vi "C37 Get PMU Real Data.vi"(7 "Array Lengths":T1, 10 "pseudoPdcId":i32, 11 "pmuIndex":i32) -> (1 "Digital Values":bool[](array[boolean]), 2 "Analog Values":sgl[](array[numeric]), 3 "Phasor Values":csg[](array[numeric]), 4 "Frequency":sgl, 5 "function return":i32, 6 "Delta Frequency":sgl)   [LabVIEW 2012]
doc: "STRONGRIDIEEEC37118DLL_API int __cdecl getPmuRealDataLabview(noArraysPmuDataFrame* rd, PmuStatus* status,\n uint16_t PhasorArrayLength, float* phasorValueReal, float* phasorValueImaginary,\n uint16_t AnalogArrayLength, float* analogValueArr,\n uint16_t DigitalArrayLength, uint8_t* digitalValueArr,\n int32_t pseudoPdcId, int32_t pmuIndex);\n\nSTRONGRIDIEEEC37118DLL_API int __cdecl getPmuRealDataLabview(noArraysPmuDataFrame* rd, PmuStatus* status,\n uint16_t PhasorArrayLength, float* phasorValueReal, float* phasorValueImaginary,\n uint16_t AnalogArrayLength, float* analogValueArr,\n uint16_t DigitalArrayLength, uint8_t* digitalValueArr,\n int32_t pseudoPdcId, int32_t pmuIndex);"
uses:
  Auto Generated/StrongridDLL.dll
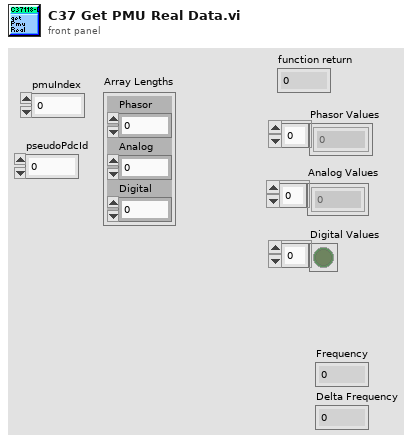
[diagram p1: front panel]
types:
  T1 = cluster{"Phasor":i32, "Analog":i32, "Digital":i32}
  T2 = cluster{"dataErrorCode":u8, "pmuSyncFlag":u8, "pmuDataSortingFlag":u8, "pmuTriggerFlag":u8, "configChangeFlag":u8, "dataModifiedFlag":u8, "timeQualityCode":u8, "unlockTimeCode":u8, "triggerReasonCode":u8}
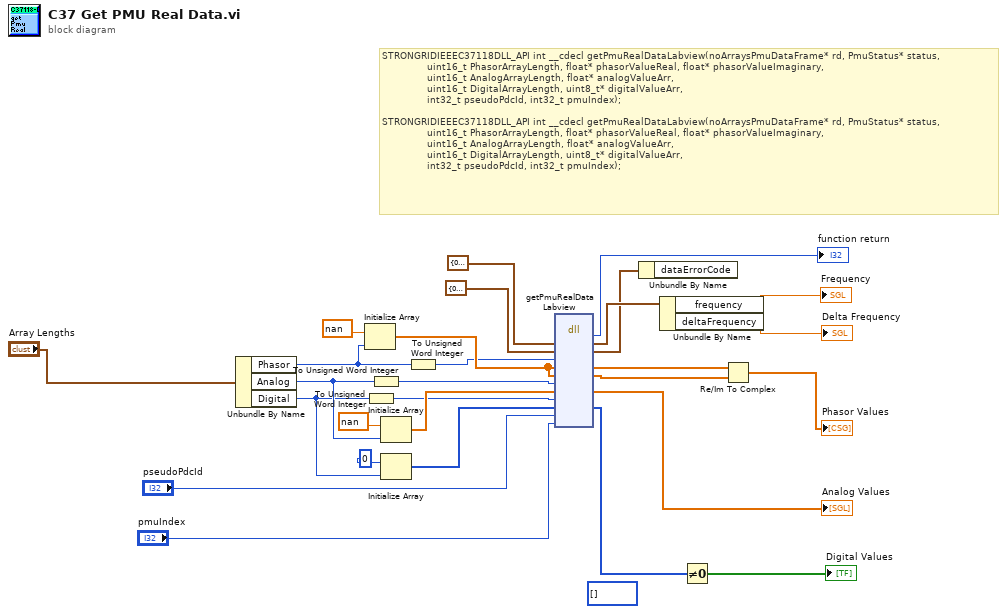
[diagram p0: block diagram]
diagram:
  (unwired) i8[] [] ("digitalValueArr")
  # "STRONGRIDIEEEC37118DLL_API int __cdecl getPmuRealDataLabview(noArraysPmuDataFrame* rd, PmuStatus* status,\n               uint16_t PhasorArrayLength, float* phasorValueReal, float* phasorValueImaginary,\n               uint16_t AnalogArrayLength, float* analogValueArr,\n               uint16_t DigitalArrayLength, uint8_t* digitalValueArr,\n               int32_t pseudoPdcId, int32_t pmuIndex);\n\nSTRONGRIDIEEEC37118DLL_API int __cdecl getPmuRealDataLabview(noArraysPmuDataFrame* rd, PmuStatus* status,\n\t\t\t\t\t\t\t\t\t\t\t\t\t\t\tuint16_t PhasorArrayLength, float* phasorValueReal, float* phasorValueImaginary,\n\t\t\t\t\t\t\t\t\t\t\t\t\t\t\tuint16_t AnalogArrayLength, float* analogValueArr,\n\t\t\t\t\t\t\t\t\t\t\t\t\t\t\tuint16_t DigitalArrayLength, uint8_t* digitalValueArr,\n\t\t\t\t\t\t\t\t\t\t\t\t\t\t\tint32_t pseudoPdcId, int32_t pmuIndex);"
  n1 = Unbundle By Name("Array Lengths") -> ("Phasor"=w12:i32, "Analog"=w8:i32, "Digital"=w5:i32)
  n2 = Initialize Array(sgl nan ("frequency"), w12) -> (w10:sgl[])
  n3 = To Unsigned Word Integer(number=w5) -> (unsigned 16bit integer=w1:u16)
  n4 = To Unsigned Word Integer(number=w8) -> (unsigned 16bit integer=w2:u16)
  n5 = Initialize Array(sgl nan ("frequency"), w8) -> (w7:sgl[])
  n6 = Initialize Array(i8 0 ("frequency"), w5) -> (w4:i8[])
  n7 = To Unsigned Word Integer(number=w12) -> (unsigned 16bit integer=w3:u16)
  n8 = dll-call lib="C:/dev/c37118-dll/labview/vi/Auto Generated/StrongridDLL.*" fn="getPmuRealDataLabview"("rd"=cluster{"frequency":sgl, "deltaFrequency":sgl} {"frequency"=0.0, "deltaFrequency"=0.0}, "status"=T2 {"dataErrorCode"=0, "pmuSyncFlag"=0, "pmuDataSortingFlag"=0, "pmuTriggerFlag"=0, "configChangeFlag"=0, "dataModifiedFlag"=0, "timeQualityCode"=0, "unlockTimeCode"=0, "triggerReasonCode"=0}, "PhasorArrayLength"=w3, "phasorValueReal"=w10, "phasorValueImaginary"=w10, "AnalogArrayLength"=w2, "analogValueArr"=w7, "DigitalArrayLength"=w1, "digitalValueArr"=w4, "pseudoPdcId"="pseudoPdcId", "pmuIndex"="pmuIndex") -> ("return type"=→"function return":i32, "rd"=w22:cluster{"frequency":sgl, "deltaFrequency":sgl}, "status"=w19:T2, "phasorValueReal"=w24:sgl[], "phasorValueImaginary"=w23:sgl[], "analogValueArr"=→"Analog Values":sgl[], "digitalValueArr"=w16:i8[])  [unwired: 8 in, 2 out]
  n9 = Unbundle By Name(w19) -> ()  [unwired: 1 out]
  n10 = Unbundle By Name(w22) -> ("frequency"=→"Frequency":sgl, "deltaFrequency"=→"Delta Frequency":sgl)
  n11 = Not Equal To 0?(x=w16) -> (x != 0?=→"Digital Values":bool[])
  n12 = Re/Im To Complex(1:w23, 2:w24) -> (0:→"Phasor Values":csg[])
